vi "PXI-Wait For Digital Trigger.vi"(0 "task in":refnum<k21>, 9 "Timeout (s)":dbl=0.5, 11 "error in (no error)":errorcluster) -> (15 "error out":errorcluster)   [LabVIEW 2020]
uses:
  <vilib>/DAQmx/read.llb/DAQmx Read (Digital Bool 1Line 1Point).vi
  <vilib>/DAQmx/miscellaneous.llb/DAQmx Fill In Error Info.vi
panel:
  in  "Poll (s)":dbl=0.001 format="%#_6p"
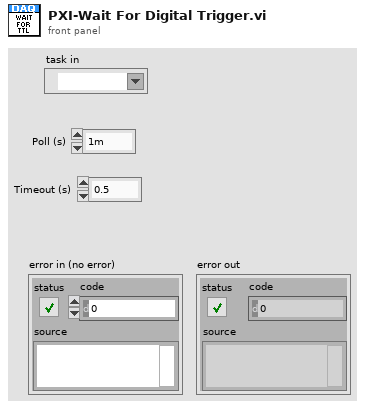
[diagram p1: front panel]
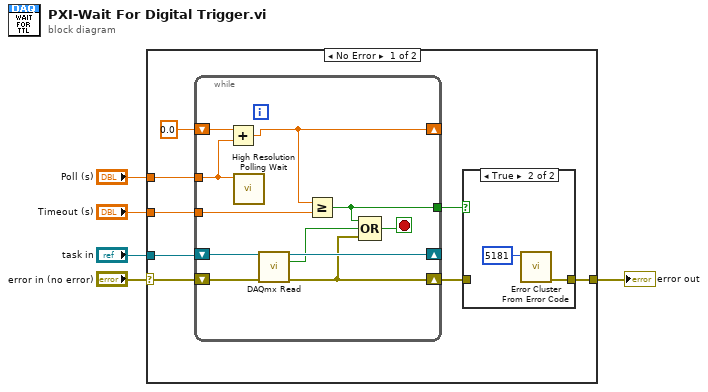
[diagram p0: block diagram]
diagram:
  n1 = case shown="No Error" "error in (no error)" {
    selector: "error in (no error)" -> [w12 w28]
    tunnel: "task in" -> [w13 _]
    tunnel: "Poll (s)" -> [w11 _]
    tunnel: [w6 w28] -> w2
    tunnel: "Timeout (s)" -> [w9 _]
    frame No Error {
      n2 = while {
        shift-right: [w18] -> w7
        shift-left: w12 -> [w25]
        shift-right: [w24] -> _
        shift-left: w13 -> [w27]
        tunnel: w11 -> [w22]
        shift-right: [w21] -> _
        shift-left: 0.0 -> [w23]
        tunnel: w9 -> [w20]
        tunnel: [w19] -> w8
        stop <- w26 stop-if-true
        n3 = Add(x=w23, y=w22) -> (x+y=w21:dbl)
        n4 = call <vilib>:"High Resolution Polling Wait.vi"("seconds to wait"=w22) -> ()  [unwired: 10 in, 1 out]
        n5 = call-poly <vilib>:"DAQmx Read.vi"("task/channels in"=w27, "error in"=w25) -> ("task out"=w24:refnum<k21>, "data"=w17:bool, "error out"=w18:errorcluster)  [unwired: 11 in]
        n6 = Greater Or Equal?(x=w21, y=w20) -> (x >= y?=w19:bool)
        n7 = Compound Arithmetic op=OR(w19, w17, w18) -> (w26:bool)
      }
      n8 = case shown="True" w8 {
        tunnel: w7 -> [w14 _]
        tunnel: [w14 w16] -> w6
        frame False {
        }
        frame True {
          n9 = call <vilib>:"Error Cluster From Error Code.vi"("error code (0)"=5181) -> ("error out"=w16:errorcluster)  [unwired: 8 in]
        }
      }
    }
    frame Error {
    }
  }
  "error out" <- w2
